vi "rs3 Advanced get AE setpoint3.vi"(8 "error in (no error)":errorcluster, 10 "mode":i32, 11 "device in":u64) -> (0 "error out 2":errorcluster, 1 "error":u64, 2 "ST_AE_Control":cluster{"meanIntensitySetpoint":u32}={"meanIntensitySetpoint"=2000}, 3 "Dev out":u64)   [LabVIEW 2017, in "libRealSense3.lvlib"]
doc: "Opens communication to a specific RealSense Device."
uses:
  libRealSense3.lvlib
  realsense2.dll
panel:
  # "RS3 Adv. Get AE Setpoint3"
  # "(C) 2017 Intel Corp.,  AGJ"
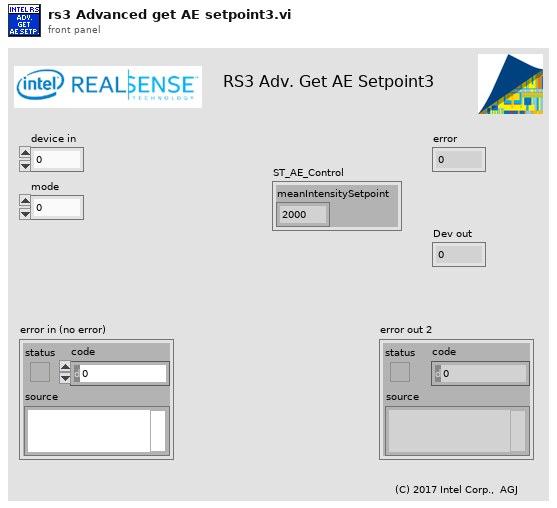
[diagram p1: front panel]
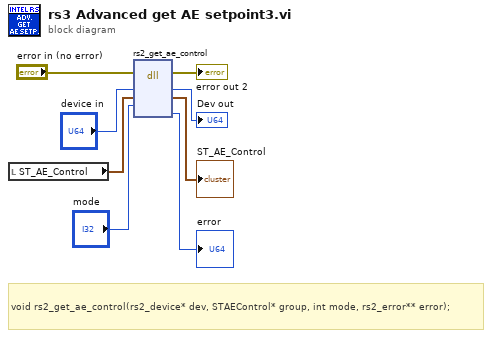
[diagram p0: block diagram]
diagram:
  # "void rs2_get_ae_control(rs2_device* dev, STAEControl* group, int mode, rs2_error** error);"
  n1 = local read "ST_AE_Control"() -> (w3:cluster{"meanIntensitySetpoint":u32})
  n2 = dll-call lib="C:/Users/agrunnet/Documents/libRealSense6/realsense2.dll" fn="rs2_get_ae_control"(error in="error in (no error)", "device"="device in", "ae control"=w3, "mode"="mode") -> (error out=→"error out 2":errorcluster, "device"=→"Dev out":u64, "ae control"=→"ST_AE_Control":cluster{"meanIntensitySetpoint":u32}, "error"=→"error":u64)  [unwired: 5 in, 1 out]
